vi "ROI from Scale Range.vi"(9 "Detail Graph Y":refnum<vi>, 10 "Detail Graph X":refnum<vi>, 11 "IntensityGraph in":refnum<vi>) -> (1 "ROI Y":cluster{"Min":i32, "Max":i32}, 2 "ROI X":cluster{"Min":i32, "Max":i32})   [LabVIEW 2023]
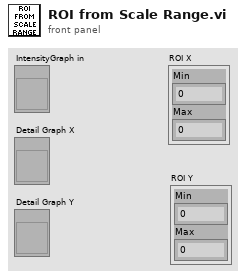
[diagram p1: front panel]
types:
  T1 = typedef "LVRangeTypeDef.ctl" = cluster{"Minimum":dbl, "Maximum":dbl, "Increment":dbl, "Minor Increment":dbl, "Start":dbl}
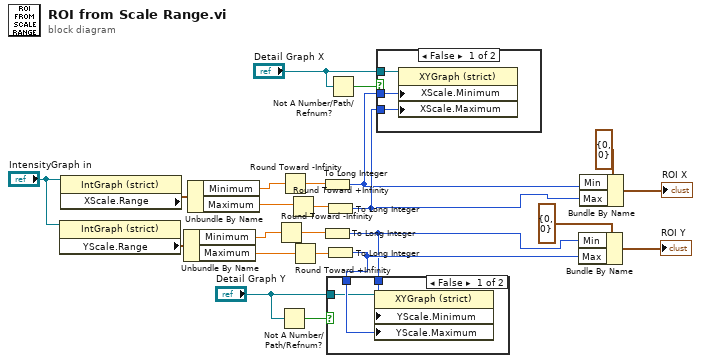
[diagram p0: block diagram]
diagram:
  n1 = property on="Property Node" class="IntGraph (strict)"(reference="IntensityGraph in") -> ("YScale.Range"=w8:T1)  [unwired: 1 in, 2 out]
  n2 = property on="Property Node" class="IntGraph (strict)"(reference="IntensityGraph in") -> ("XScale.Range"=w9:T1)  [unwired: 1 in, 2 out]
  n3 = Unbundle By Name(w8) -> ("Minimum"=w21:dbl, "Maximum"=w18:dbl)
  n4 = Unbundle By Name(w9) -> ("Minimum"=w16:dbl, "Maximum"=w14:dbl)
  n5 = Round Toward -Infinity(1:w21) -> (0:w20:dbl)
  n6 = Not A Number/Path/Refnum?(number/path/refnum="Detail Graph Y") -> (NaN/Path/Refnum?=w4:bool)
  n7 = Round Toward -Infinity(1:w16) -> (0:w17:dbl)
  n8 = Round Toward +Infinity(x=w14) -> (ceil(x): smallest int >= x=w15:dbl)
  n9 = Round Toward +Infinity(x=w18) -> (ceil(x): smallest int >= x=w19:dbl)
  n10 = To Long Integer(number=w17) -> (32bit integer=w13:i32)
  n11 = To Long Integer(number=w20) -> (32bit integer=w12:i32)
  n12 = To Long Integer(number=w15) -> (32bit integer=w23:i32)
  n13 = To Long Integer(number=w19) -> (32bit integer=w22:i32)
  n14 = case shown="False" w4 {
    tunnel: w22 -> [w26 _]
    tunnel: w12 -> [w25 _]
    tunnel: "Detail Graph Y" -> [w24 _]
    frame False {
      n15 = property on="Property Node" class="XYGraph (strict)"(reference=w24, "YScale.Minimum"=w25, "YScale.Maximum"=w26) -> ()  [unwired: 1 in, 2 out]
    }
    frame True {
    }
  }
  n16 = Not A Number/Path/Refnum?(number/path/refnum="Detail Graph X") -> (NaN/Path/Refnum?=w2:bool)
  n17 = case shown="False" w2 {
    tunnel: w23 -> [w29 _]
    tunnel: w13 -> [w28 _]
    tunnel: "Detail Graph X" -> [w27 _]
    frame False {
      n18 = property on="Property Node" class="XYGraph (strict)"(reference=w27, "XScale.Minimum"=w28, "XScale.Maximum"=w29) -> ()  [unwired: 1 in, 2 out]
    }
    frame True {
    }
  }
  n19 = Bundle By Name(cluster=cluster{"Min":i32, "Max":i32} {"Min"=0, "Max"=0} ("Y"), "Min"=w12, "Max"=w22) -> (→"ROI Y":cluster{"Min":i32, "Max":i32})
  n20 = Bundle By Name(cluster=cluster{"Min":i32, "Max":i32} {"Min"=0, "Max"=0} ("X"), "Min"=w13, "Max"=w23) -> (→"ROI X":cluster{"Min":i32, "Max":i32})
